vi "Actor-Caller.vi"(5 "Initialize-Error Passback":refnum<notifier>, 7 "Enqueuers Passback":refnum<notifier>, 8 "Owner":refnum<vi>, 9 "Did Stop Enqueuer":refnum<user-event>, 10 "Launch":refnum<notifier>, 11 "Actor in":refnum<class "Actor.lvclass">) -> ()   [LabVIEW 2018, in "Scripting.lvlib" / "Actor.lvclass"]
uses:
  Actor.lvclass
  All-Enqueuers.ctl
  Broadcast Enqueuers.ctl
  Did Initialize.ctl
  Request-Enqueuers.ctl
  Get State.ctl
  State.ctl
  Stop.ctl
  Did Stop.ctl
  Front-Panel State.ctl
  Launch.ctl
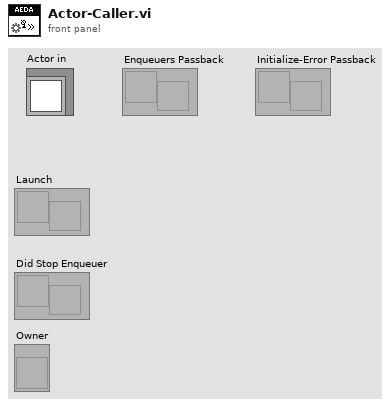
[diagram p1: front panel]
types:
  T1 = typedef "Scripting.lvlib/Actor.lvclass/Launch.ctl" = cluster{"Owner":refnum<vi>}
  T2 = typedef "Scripting.lvlib/Actor.lvclass/All-Enqueuers.ctl" = cluster{"Broadcasts":T3, "Requests":T4}
  T3 = typedef "Scripting.lvlib/Actor.lvclass/Broadcast Enqueuers.ctl" = cluster{"Did Initialize":refnum<user-event>}
  T4 = typedef "Scripting.lvlib/Actor.lvclass/Request-Enqueuers.ctl" = cluster{"Get State":refnum<user-event>, "Stop":refnum<user-event>}
  T5 = typedef "Scripting.lvlib/Actor.lvclass/Did Stop.ctl" = cluster{"State":refnum<class "Actor.lvclass">, "Final Error":errorcluster}
  T6 = typedef "Scripting.lvlib/Actor.lvclass/API-Requests.ctl" = refnum<event-registration>
  T7 = typedef "Scripting.lvlib/Actor.lvclass/Front-Panel State.ctl" = enum16{"Don't Show", "Show"}
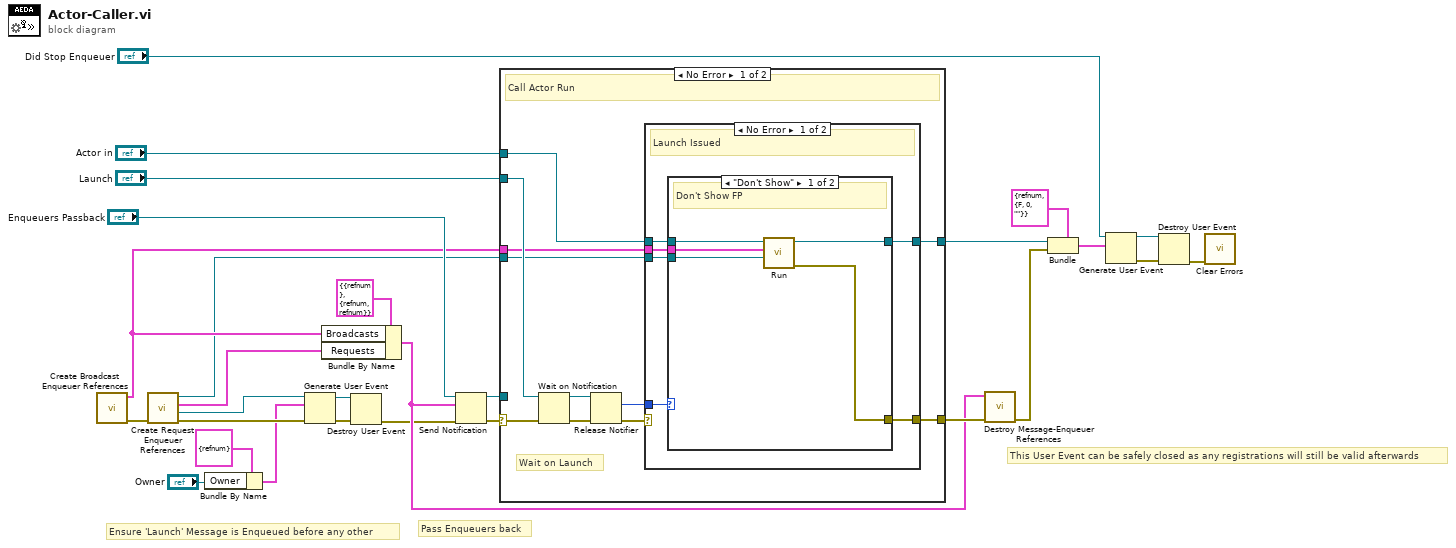
[diagram p0: block diagram]
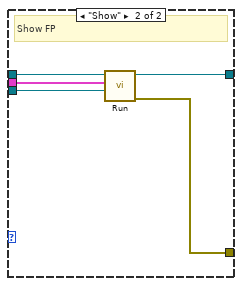
[diagram p2: hidden frame]
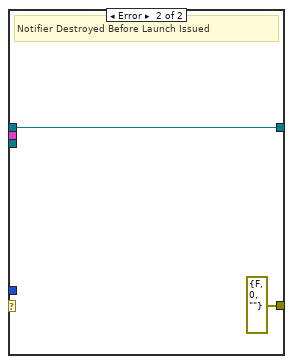
[diagram p3: hidden frame]
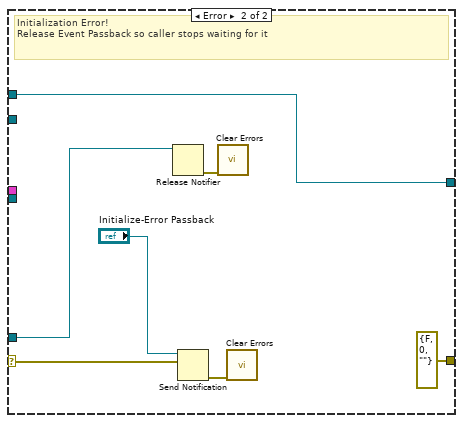
[diagram p4: hidden frame]
diagram:
  # "Ensure 'Launch' Message is Enqueued before any other"
  # "This User Event can be safely closed as any registrations will still be valid afterwards"
  # "Pass Enqueuers back"
  n1 = call "Create Broadcast Enqueuer References.vi"() -> ("error out"=w12:errorcluster, "Broadcasts"=w13:T3)  [unwired: 10 in]
  n2 = call "Create Request Enqueuer References.vi"("error in (no error)"=w12) -> ("error out"=w11:errorcluster, "Launch Enqueuer"=w7:refnum<user-event>, "Request-Enqueuers"=w2:T4, "API-Requests"=w3:T6)  [unwired: 7 in]
  n3 = Bundle By Name(cluster=T1 {"Owner"=refnum} ("event data"), "Owner"="Owner") -> (w1:T1)
  n4 = Generate User Event(user event=w7, event data cluster=w1, error in=w11) -> (user event out=w6:refnum<user-event>, error out=w5:errorcluster)  [unwired: 1 in]
  n5 = Bundle By Name(cluster=T2 {"Broadcasts"={"Did Initialize"=refnum}, "Requests"={"Get State"=refnum, "Stop"=refnum}} ("Enqueuers"), "Broadcasts"=w13, "Requests"=w2) -> (w8:T2)
  n6 = Destroy User Event(user event=w6, error in=w5) -> (error out=w4:errorcluster)
  n7 = Send Notification(notification=w8, notifier="Enqueuers Passback", error in (no error)=w4) -> (notifier out=w20:refnum<notifier>, error out=w24:errorcluster)
  n8 = case shown="No Error" w24 {
    selector: w24 -> [w37 w60]
    tunnel: "Launch" -> [w39 _]
    tunnel: "Actor in" -> [w38 w64]
    tunnel: [w31 errorcluster {"status"=FALSE, "code"=0, "source"=""} ("error out")] -> w19
    tunnel: [w36 w64] -> w21
    tunnel: w20 -> [_ w63]
    tunnel: w13 -> [w30 _]
    tunnel: w3 -> [w29 _]
    frame No Error {
      # "Wait on Launch"
      # "Call Actor Run"
      n9 = Wait on Notification(notifier=w39, error in (no error)=w37) -> (notifier out=w34:refnum<notifier>, error out=w35:errorcluster)  [unwired: 2 in, 2 out]
      n10 = Release Notifier(notifier=w34, error in (no error)=w35) -> (last notification=w33:T7, error out=w32:errorcluster)  [unwired: 1 in, 1 out]
      n11 = case shown="No Error" w32 {
        tunnel: w38 -> [w45 w57]
        tunnel: [w44 w57] -> w36
        tunnel: [w43 errorcluster {"status"=FALSE, "code"=0, "source"=""} ("error out")] -> w31
        tunnel: w33 -> [w42 _]
        tunnel: w30 -> [w41 _]
        tunnel: w29 -> [w40 _]
        frame No Error {
          # "Launch Issued"
          n12 = case shown="\"Don't Show\"" w42 {
            tunnel: w45 -> [w50 w55]
            tunnel: [w49 w53] -> w43
            tunnel: [w48 w54] -> w44
            tunnel: w41 -> [w47 w52]
            tunnel: w40 -> [w46 w51]
            frame "Don't Show" {
              # "Don't Show FP"
              n13 = call-dynamic "Run.vi"("API-Requests"=w46, "Broadcast-Enqueuers"=w47, "Actor in"=w50) -> ("error out"=w49:errorcluster, "Actor out"=w48:refnum<class "Actor.lvclass">)  [unwired: 7 in]
            }
            frame "Show" {
              # "Show FP"
              n14 = call-dynamic "Run.vi"("API-Requests"=w51, "Broadcast-Enqueuers"=w52, "Actor in"=w55) -> ("error out"=w53:errorcluster, "Actor out"=w54:refnum<class "Actor.lvclass">)  [unwired: 7 in]
            }
          }
        }
        frame Error {
          # "Notifier Destroyed Before Launch Issued"
        }
      }
    }
    frame Error {
      # "Initialization Error!\nRelease Event Passback so caller stops waiting for it"
      n15 = Release Notifier(notifier=w63) -> (error out=w62:errorcluster)  [unwired: 2 in, 2 out]
      n16 = Send Notification(notification=w60, notifier="Initialize-Error Passback") -> (error out=w59:errorcluster)  [unwired: 1 in, 1 out]
      n17 = call <vilib>:"Clear Errors.vi"("error in (no error)"=w62) -> ()  [unwired: 5 in, 2 out]
      n18 = call <vilib>:"Clear Errors.vi"("error in (no error)"=w59) -> ()  [unwired: 5 in, 2 out]
    }
  }
  n19 = call "Destroy Message-Enqueuer References.vi"("error in (no error)"=w19, "Event-References"=w8) -> ("error out"=w18:errorcluster)  [unwired: 9 in]
  n20 = Bundle(cluster=T5 {"State"=refnum, "Final Error"={"status"=FALSE, "code"=0, "source"=""}} ("event data"), "State"=w21, "Final Error"=w18) -> (w28:T5)
  n21 = Generate User Event(user event="Did Stop Enqueuer", event data cluster=w28) -> (user event out=w17:refnum<user-event>, error out=w16:errorcluster)  [unwired: 2 in]
  n22 = Destroy User Event(user event=w17, error in=w16) -> (error out=w15:errorcluster)
  n23 = call <vilib>:"Clear Errors.vi"("error in (no error)"=w15) -> ()  [unwired: 5 in, 2 out]
